vi "Current to DAC code.vi"(1 "Galv. cal. data":dbl[][](array[numeric]), 2 "Current Range":string, 3 "DAC output (µA)":dbl) -> (0 "Code out":u16)   [LabVIEW 2015]
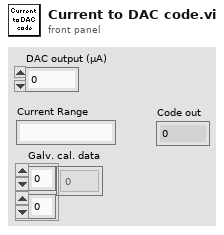
[diagram p1: front panel]
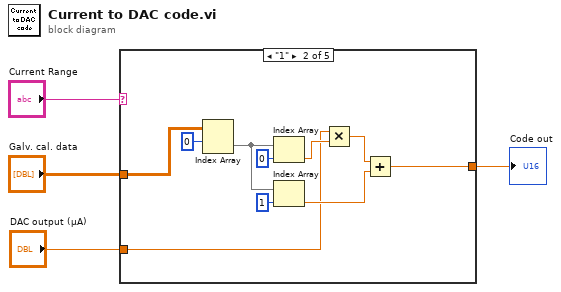
[diagram p0: block diagram]
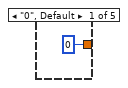
[diagram p2: hidden frame]
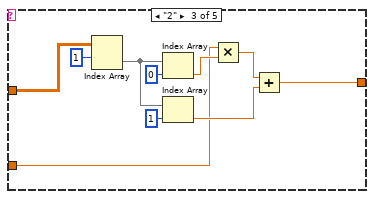
[diagram p3: hidden frame]
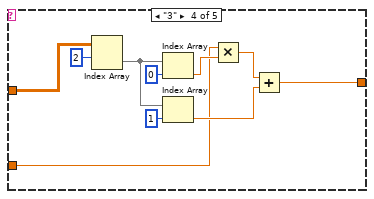
[diagram p4: hidden frame]
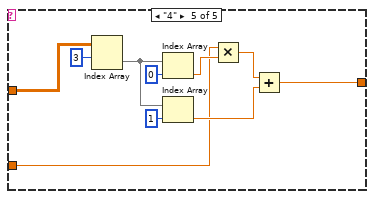
[diagram p5: hidden frame]
diagram:
  n1 = case shown="\"1\"" "Current Range" {
    tunnel: "Galv. cal. data" -> [_ w15 w25 w35 w45]
    tunnel: "DAC output (µA)" -> [_ w7 w17 w27 w37]
    tunnel: [u16 0 w6 w16 w26 w36] -> w2
    frame "0", Default {
    }
    frame "1" {
      n2 = Index Array(array=w15, index (row)=0 ("index")) -> (element=w11:dbl[])  [unwired: 1 in]
      n3 = Index Array(array=w11, index=0) -> (element=w10:dbl)
      n4 = Index Array(array=w11, index=1) -> (element=w9:dbl)
      n5 = Multiply(x=w7, y=w10) -> (x*y=w8:dbl)
      n6 = Add(x=w8, y=w9) -> (x+y=w6:dbl)
    }
    frame "2" {
      n7 = Index Array(array=w25, index (row)=1 ("index")) -> (element=w21:dbl[])  [unwired: 1 in]
      n8 = Index Array(array=w21, index=0) -> (element=w20:dbl)
      n9 = Index Array(array=w21, index=1) -> (element=w19:dbl)
      n10 = Multiply(x=w17, y=w20) -> (x*y=w18:dbl)
      n11 = Add(x=w18, y=w19) -> (x+y=w16:dbl)
    }
    frame "3" {
      n12 = Index Array(array=w35, index (row)=2 ("index")) -> (element=w31:dbl[])  [unwired: 1 in]
      n13 = Index Array(array=w31, index=0) -> (element=w30:dbl)
      n14 = Index Array(array=w31, index=1) -> (element=w29:dbl)
      n15 = Multiply(x=w27, y=w30) -> (x*y=w28:dbl)
      n16 = Add(x=w28, y=w29) -> (x+y=w26:dbl)
    }
    frame "4" {
      n17 = Index Array(array=w45, index (row)=3 ("index")) -> (element=w41:dbl[])  [unwired: 1 in]
      n18 = Index Array(array=w41, index=0) -> (element=w40:dbl)
      n19 = Index Array(array=w41, index=1) -> (element=w39:dbl)
      n20 = Multiply(x=w37, y=w40) -> (x*y=w38:dbl)
      n21 = Add(x=w38, y=w39) -> (x+y=w36:dbl)
    }
  }
  "Code out" <- w2
